vi "NML Multi Oscilloscope.vi"() -> ()   [LabVIEW 2020]
doc: "This VI is designed to scan data from several A/D channels. The first channel is converted to Tesla using the magnet ID (or 'None' for volts). The channels are scanned at an interval of 250µSec/Channel. The minimum interval between scans is 1mSec.\nScott Hannahs, FBNML, April 1992"
uses:
  Sub Controls/Magnet List.ctl
  Sub Controls/Gain Selector.ctl
panel:
  out "Data":dbl[][](array[numeric]) format="%.2f"
  in  "?":dbl[](array[numeric])=[1.0, 1.0, 1.0, 1.0, 1.0, 1.0, 1.0, 1.0] format="%.1e"
  in  "RANGE & CHANNEL SELECTOR":T2={"0"=3, "1"=1, "2"=0, "3"=0, "4"=0, "5"=0, "6"=0, "7"=0} {"7" scale=0.0..4.0; "6" scale=0.0..4.0; "5" scale=0.0..4.0; "4" scale=0.0..4.0; "3" scale=0.0..4.0; "2" scale=0.0..4.0; "1" scale=0.0..4.0; "0" scale=0.0..4.0}
  in  "ÆT (msec)":sgl=10.0 min=0.1 format="%.2f"
  in  "# Points":i32=1000 min=3 max=32000
  in  "Bipolar":bool
  in  "New":bool
  out "COLLECTING":bool
  in  "Magnet ID":T3 items=["None", "SCM1", "SCM2", "Cell 3", "Cell 4", "Cell 5", "Cell 6", "Cell 7", "Cell 8", "Cell 9", "Cell 12"]
  in  "Column for X-Axis":i32(ring) items=["Point #", "Field", "Column 2", "Column 3", "Column 4", "Column 5", "Column 6", "Column 7", "Column 8", "Column 9", "Column 10"]
  in  "Display?":bool[](array[boolean])=[FALSE, FALSE, FALSE, FALSE, FALSE, FALSE, FALSE, FALSE, FALSE, FALSE, FALSE, FALSE, FALSE, FALSE, FALSE, FALSE, FALSE]
  out "File Error:":string
  in  "Magnet List":string="None\r1F\r1G\r1K\r1L\r1M\r1P\r1Za Hybrid\r1Za Insert\r1Za 1000A\r1Zb Hybrid\r1Zb Insert\r1Zb 1000A\r1Zc Hybrid\r1Zc Insert\r1Zc 1000A\r2B\r2F\r2G\r2H\r2I\r2K\r2L\r2M\r2P\r2R\r2S\r2T\r2U\r2V\r2W\r2X\r2Y\r2Za Hybrid\r2Za Insert\r2Za 1000A\r2Zb Hybrid\r2Zb Insert\r2Zb 1000A\r2Zc Hybrid\r2Zc Insert\r2Zc 1000A\r4B4\r4D\r6B\r10A\rHybrid Supercon\rSupercon\r"
  out "?":cluster{dbl[], dbl[]}[](graph)
  out "Calibration Error":string
  in  "Comments":string="This data's for you."
  in  "User Name":string="Conan the SCIENTIST"
  in  "File":string="Test"
  # "Monopolar"
  # "Field [tesla]"
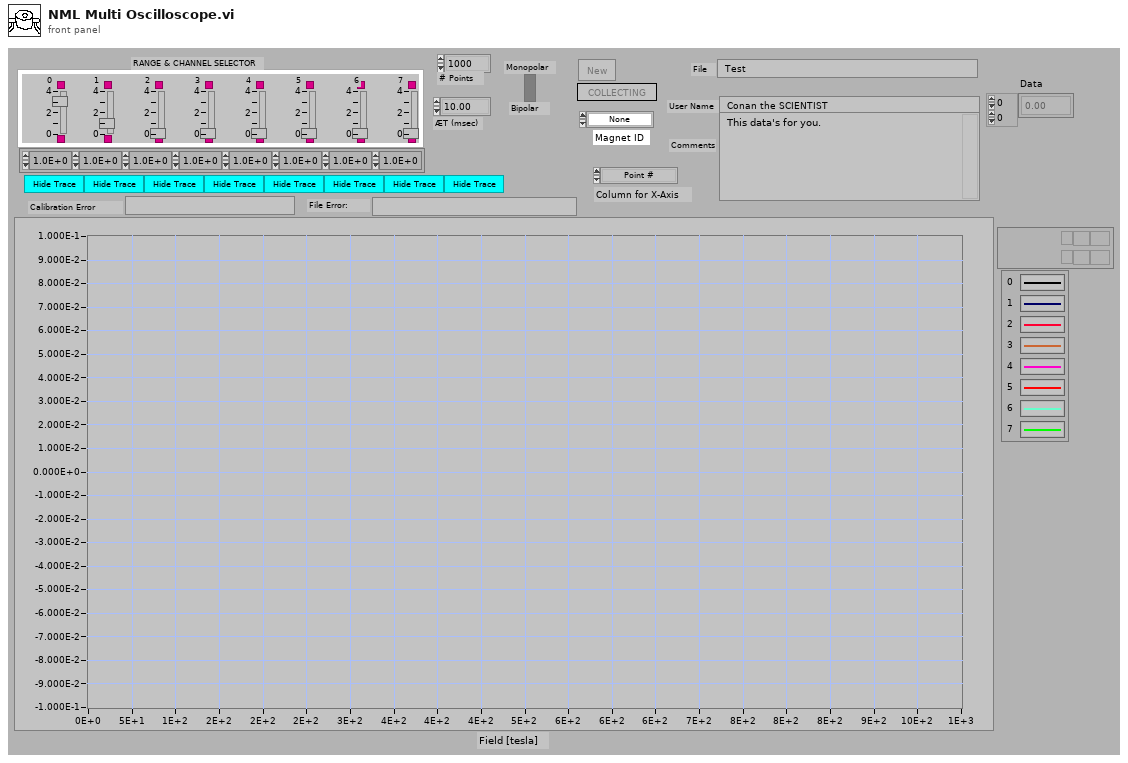
[diagram p1: front panel]
types:
  T1 = typedef "Gain Selector.ctl" = i16
  T2 = cluster{"0":T1, "1":T1, "2":T1, "3":T1, "4":T1, "5":T1, "6":T1, "7":T1}
  T3 = typedef "Magnet List.ctl" = i32
  T4 = cluster{"Current Scale Factor kA/V":dbl, "I->B":dbl[], "B->I":dbl[]}
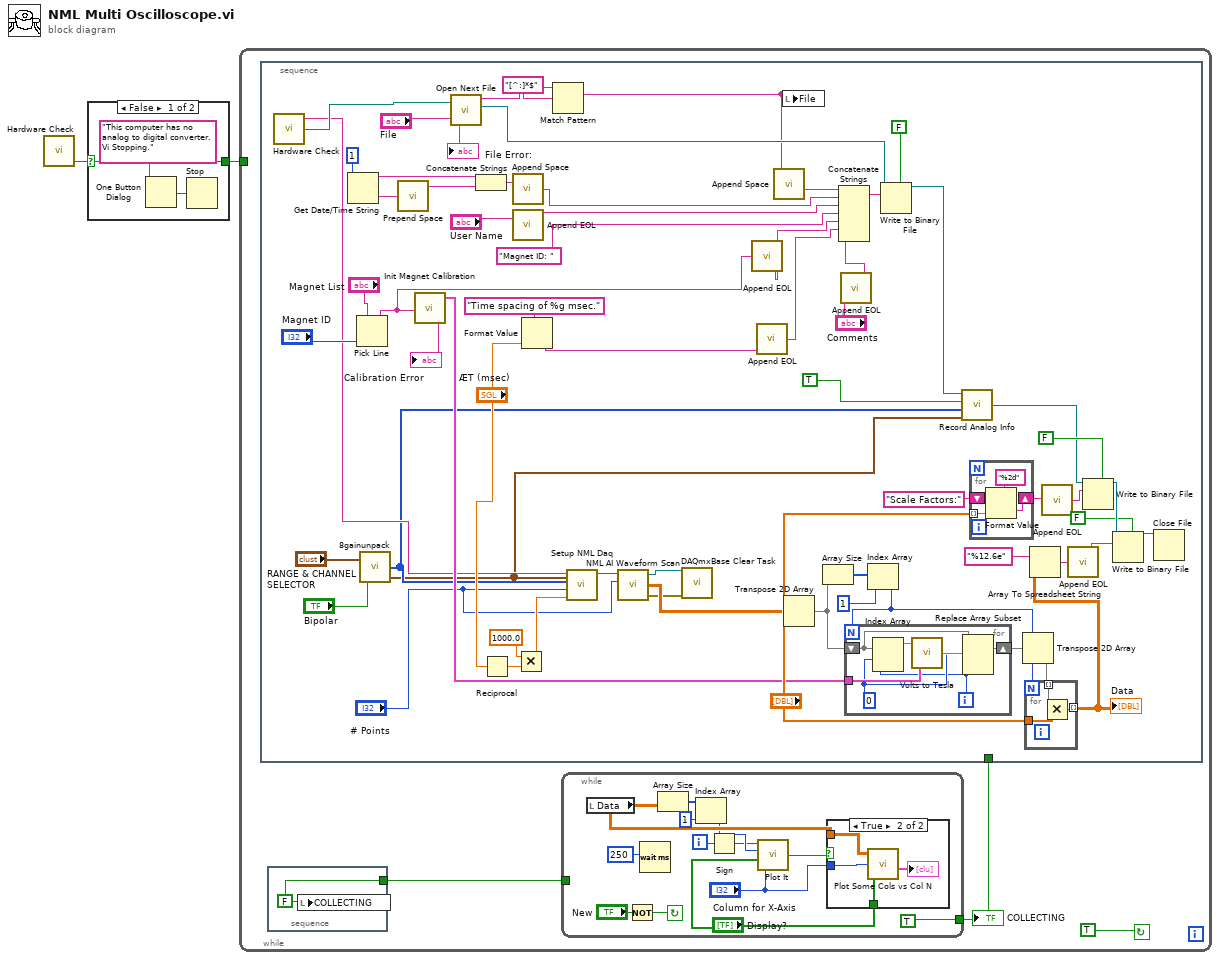
[diagram p0: block diagram]
diagram:
  n1 = call "Hardware Check.vi"() -> ("Has A/D board"=w2:bool)  [unwired: 1 in, 2 out]
  n2 = case shown="False" w2 {
    selector: w2 -> [w3 w6]
    tunnel: [w3 w6] -> w1
    frame False {
      n3 = One Button Dialog(message="This computer has no analog to digital converter.  Vi Stopping.") -> (true=w4:bool)  [unwired: 1 in]
      n4 = Stop(stop? (T)=w4) -> ()
    }
    frame True {
    }
  }
  n5 = while {
    tunnel: w1 -> [_]
    stop <- TRUE continue-if-true
    n6 = stacked-sequence {
      tunnel: [w27] -> w7
      frame #0 {
        w27 = FALSE
        n7 = local write "COLLECTING"(w27) -> ()
      }
    }
    n8 = while {
      tunnel: w7 -> [_]
      tunnel: [TRUE] -> w8
      i -> [w19]
      stop <- w22 continue-if-true
      n9 = local read "Data"() -> (w17:dbl[][])
      n10 = Not(x="New") -> (.not. x?=w22:bool)
      n11 = Wait (ms)(milliseconds to wait=u32 250) -> ()  [unwired: 1 out]
      n12 = Array Size(array=w17) -> (size(s)=w15:i32[])
      n13 = Index Array(array=w15, index=1) -> (element=w13:i32)
      n14 = Sign(1:w19) -> (0:w12:i32)
      n15 = call "Plot It.vi"("X-Axis"="Column for X-Axis", "Display?"="Display?", "# of columns"=w13, "Index"=w12) -> (0:w20:bool)
      n16 = case shown="True" w20 {
        tunnel: "Display?" -> [_ w26]
        tunnel: w17 -> [_ w24]
        tunnel: "Column for X-Axis" -> [_ w23]
        frame False {
        }
        frame True {
          n17 = call "Plot Some Cols vs Col N.vi"("Display/hide"=w26, "Column for abscissa"=w23, "Input Array"=w24) -> ("Output Graph"=→"?":cluster{dbl[], dbl[]}[])
        }
      }
    }
    "COLLECTING" <- w8
    n18 = stacked-sequence {
      tunnel: w8 -> [_]
      frame #0 {
        # "Magnet Calibration Coefficents"
        n19 = call "Hardware Check.vi"() -> ("Data Acq Device"=w39:string, "Data Directory Path"=w89:path)  [unwired: 1 in, 1 out]
        n20 = Get Date/Time String(date format (0)=1) -> (date string=w63:string, time string=w65:string)  [unwired: 2 in]
        n21 = Pick Line(multi-line string="Magnet List", line index="Magnet ID") -> (output string=w72:string)  [unwired: 1 in]
        n22 = call "8gainunpack.vi"("GAIN & CHANNEL SELECTOR"="RANGE & CHANNEL SELECTOR", "Monopolar"="Bipolar") -> ("channels (0)"=w30:i32[], "Input Limits"=w29:cluster{"High Limit":dbl, "Low Limit":dbl}[])  [unwired: 1 out]
        n23 = call "Prepend Space.vi"("Input String"=w65) -> ("Space + Input String"=w64:string)
        n24 = call "Init Magnet Calibration.vi"("Magnet Id"=w72) -> ("Calibration"=w52:T4, "Error message"=→"Calibration Error":string)  [unwired: 1 out]
        n25 = call "Open Next File.vi"("Input File Pattern"="File", "Dir Path"=w89) -> ("Error Message"=→"File Error:":string, "File Ref Num"=w71:refnum<file>, "Output File Name"=w74:string)  [unwired: 1 in, 1 out]
        n26 = Concatenate Strings(w63, w64) -> (w62:string)
        n27 = Reciprocal(x="ÆT (msec)") -> (1/x=w86:sgl)
        n28 = call "Append Space.vi"("INPUT STRING"=w62) -> ("OUTPUT STRING (PLUS [SPACE])"=w57:string)
        n29 = call "Append EOL.vi"("INPUT STRING"="User Name") -> ("OUTPUT STRING (PLUS End of Line)"=w58:string)
        n30 = Multiply(x=sgl 1000.0, y=w86) -> (x*y=w37:sgl)
        n31 = Format Value(format string="Time spacing of %g msec.", value (0)="ÆT (msec)") -> (output string=w55:string)  [unwired: 1 in]
        n32 = Match Pattern(string=w74, regular expression="[^:]*$") -> (match substring=w44:string)  [unwired: 1 in, 3 out]
        n33 = call "Setup NML Daq.vi"("Input Limits"=w29, "rate"=w37, "number of samples per channel"="# Points", "channels (0)"=w30, "Data Acq Device"=w39) -> ("task out"=w38:refnum<k21>)  [unwired: 5 in, 1 out]
        n34 = call "NML AI Waveform Scan.vi"("task/channels in"=w38, "Number to Average"="# Points") -> ("task out"=w34:refnum<k21>, "Scaled data"=w36:dbl[][], "error out"=w33:errorcluster)  [unwired: 4 in]
        n35 = call <vilib>:"DAQmxBase Clear Task.vi"("task in"=w34, "error in"=w33) -> ()  [unwired: 13 in, 1 out]
        n36 = call "Append EOL.vi"("INPUT STRING"=w72) -> ("OUTPUT STRING (PLUS End of Line)"=w60:string)
        n37 = call "Append EOL.vi"("INPUT STRING"=w55) -> ("OUTPUT STRING (PLUS End of Line)"=w67:string)
        n38 = call "Append Space.vi"("INPUT STRING"=w44) -> ("OUTPUT STRING (PLUS [SPACE])"=w56:string)
        n39 = local write "File"(w44) -> ()
        n40 = Transpose 2D Array(2D array=w36) -> (transposed array=w85:dbl[][])
        n41 = Array Size(array=w85) -> (size(s)=w78:i32[])
        n42 = call "Append EOL.vi"("INPUT STRING"="Comments") -> ("OUTPUT STRING (PLUS End of Line)"=w61:string)
        n43 = Concatenate Strings(w56, w57, w58, "Magnet ID: ", w60, w67, w61) -> (w53:string)
        n44 = Index Array(array=w78, index=1) -> (element=w80:i32)
        n45 = for {
          N: w80 -> [_]
          shift-right: [w101] -> w81
          shift-left: w85 -> [w100]
          tunnel: w52 -> [w105]
          i -> [w103]
          w104 = 0
          n46 = Index Array(array=w100, index (row)=w104, index (col)=w103) -> (element=w102:dbl)
          n47 = call "Volts to Tesla.vi"("Calibration"=w105, "Console voltage"=w102) -> ("Field"=w106:dbl)
          n48 = Replace Array Subset(array=w100, new element=w106, index (row)=w104, index (col)=w103) -> (w101:dbl[][])
        }
        n49 = Write to Binary File(file (use dialog)=w71, data=w53, 5:FALSE ("prepend array or string size? (T)")) -> (refnum out=w32:refnum<file>)  [unwired: 3 in, 2 out]
        n50 = call "Record Analog Info.vi"("input limits (no change)"=w29, "channels (0)"=w30, "Boolean"=TRUE, "File Ref Num 2"=w32) -> ("File Ref Num"=w28:refnum<file>)
        n51 = for {
          shift-right: [w96] -> w69
          shift-left: "Scale Factors:" -> [w94]
          tunnel: "?" -> [w93] mode=indexing
          n52 = Format Value(string ("")=w94, format string="%2d", value (0)=w93) -> (output string=w96:string)
        }
        n53 = Transpose 2D Array(2D array=w81) -> (transposed array=w77:dbl[][])
        n54 = for {
          N: w80 -> [_]
          tunnel: [w97] -> w76 mode=indexing
          tunnel: w77 -> [w98] mode=indexing
          tunnel: "?" -> [w99]
          n55 = Multiply(x=w98, y=w99) -> (x*y=w97:dbl[])
        }
        "Data" <- w76
        n56 = Array To Spreadsheet String(array=w76, 3:"%12.6e") -> (spreadsheet string=w84:string)  [unwired: 1 in]
        n57 = call "Append EOL.vi"("INPUT STRING"=w69) -> ("OUTPUT STRING (PLUS End of Line)"=w68:string)
        n58 = call "Append EOL.vi"("INPUT STRING"=w84) -> ("OUTPUT STRING (PLUS End of Line)"=w82:string)
        n59 = Write to Binary File(file (use dialog)=w28, data=w68, 5:FALSE ("prepend array or string size? (T)")) -> (refnum out=w51:refnum<file>)  [unwired: 3 in, 2 out]
        n60 = Write to Binary File(file (use dialog)=w51, data=w82, 5:FALSE ("prepend array or string size? (T)")) -> (refnum out=w75:refnum<file>)  [unwired: 3 in, 2 out]
        n61 = Close File(refnum=w75) -> ()  [unwired: 1 in, 2 out]
      }
    }
  }
